vi "Create Node.vi"(8 "error in (no error)":errorcluster, 10 "UID":string, 11 "Base Tree in":refnum<class "Base Tree.lvclass">) -> (0 "error out":errorcluster, 3 "Base Tree out":refnum<class "Base Tree.lvclass">)   [LabVIEW 2017, in "Browser Core.lvlib" / "Base Tree.lvclass"]
doc: "Create new Node and Add to Tree dictionary"
uses:
  Base Tree.lvclass
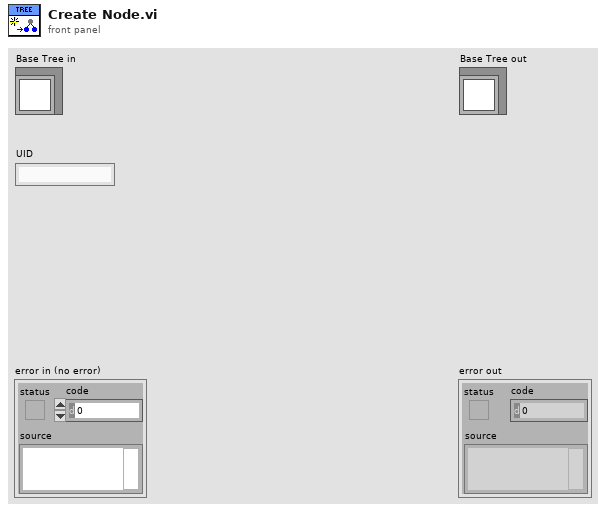
[diagram p1: front panel]
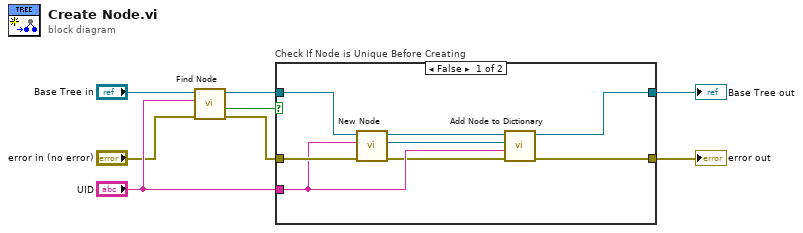
[diagram p0: block diagram]
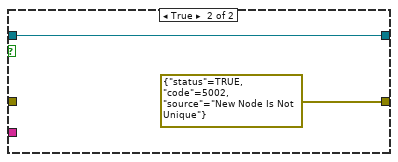
[diagram p2: hidden frame]
diagram:
  n1 = call-dynamic "Find Node.vi"("error in (no error)"="error in (no error)", "UID"="UID", "Base Tree in"="Base Tree in") -> ("error out"=w4:errorcluster, "Found?"=w5:bool, "Base Tree out"=w3:refnum<class "Base Tree.lvclass">)  [unwired: 4 in, 2 out]
  n2 = case "Check If Node is Unique Before Creating" shown="False" w5 {
    tunnel: "UID" -> [w12 _]
    tunnel: w4 -> [w15 _]
    tunnel: w3 -> [w14 w17]
    tunnel: [w11 errorcluster {"status"=TRUE, "code"=5002, "source"="New Node Is Not Unique"} ("error out")] -> w2
    tunnel: [w10 w17] -> w1
    frame False {
      n3 = call-dynamic "New Node.vi"("error in (no error)"=w15, "UID"=w12, "Base Tree in"=w14) -> ("error out"=w11:errorcluster, "Generic Node out"=w9:refnum<class "Generic Node.lvclass">, "Base Tree out"=w13:refnum<class "Base Tree.lvclass">)  [unwired: 6 in]
      n4 = call "Add Node to Dictionary.vi"("Error In"=w11, "UID"=w12, "New Node"=w9, "Base Tree in"=w13) -> ("Base Tree out"=w10:refnum<class "Base Tree.lvclass">)  [unwired: 7 in]
    }
    frame True {
    }
  }
  "error out" <- w2
  "Base Tree out" <- w1
